vi "Stop Dependency.vi"(4 "timeout in ms (-1)":i32=-1, 6 "Destroy ref? (T)":bool=TRUE, 8 "error in (no error)":errorcluster, 9 "Name (ignored if reference valid)":string, 10 "Dependency Reference":refnum<class "SMO.lvclass">, 11 "SMO in":refnum<class "SMO.lvclass">) -> (0 "error out":errorcluster, 2 "Dependency Reference out":refnum<class "SMO.lvclass">, 3 "SMO out":refnum<class "SMO.lvclass">)   [LabVIEW 2021, in "smo.lvlib" / "SMO.lvclass"]
uses:
  SMO.lvclass
  SMO.lvclass/SMO.ctl
  Support/Attribute.Owner/Attribute.Owner.lvclass
  Typedefs/SMO Dependency Event--Enum.ctl
  Typedefs/SMO Dependency Event--Cluster.ctl
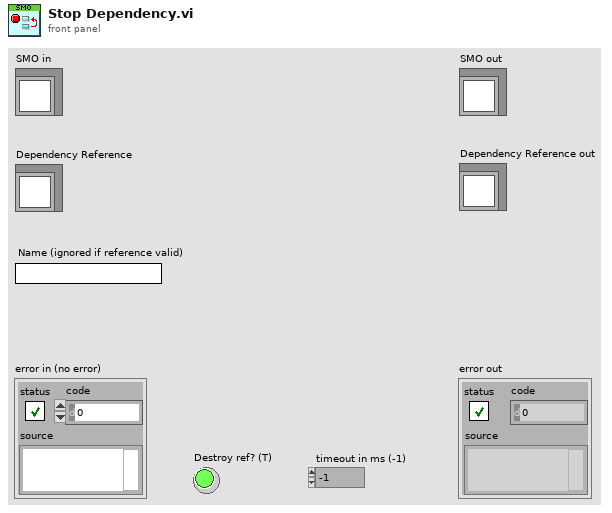
[diagram p1: front panel]
types:
  T1 = typedef "smo.lvlib/SMO.lvclass/SMO Dependency Event--Cluster.ctl" = cluster{"Name":string, "GUID":string, "Event":T2}
  T2 = typedef "smo.lvlib/SMO.lvclass/SMO Dependency Event--Enum.ctl" = enum16{"Added", "Removed", "Started", "Stopped"}
  T3 = typedef "smo.lvlib/SMO.lvclass/Protected Events.ctl" = cluster{"StopProcesses":refnum<user-event>, "AbortProcesses":refnum<user-event>, "Config Changed":refnum<user-event>, "Dependency":refnum<user-event>}
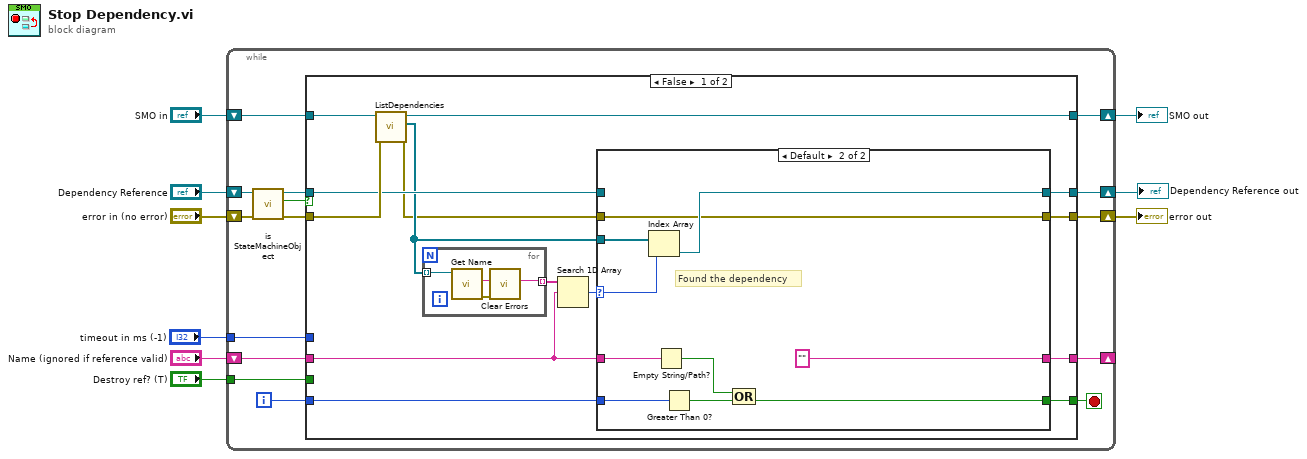
[diagram p0: block diagram]
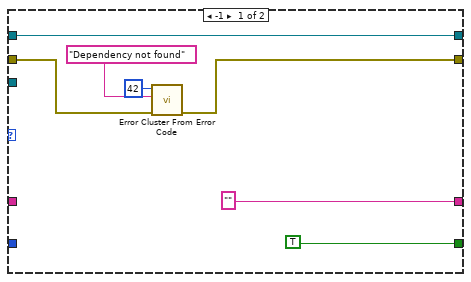
[diagram p2: hidden frame]
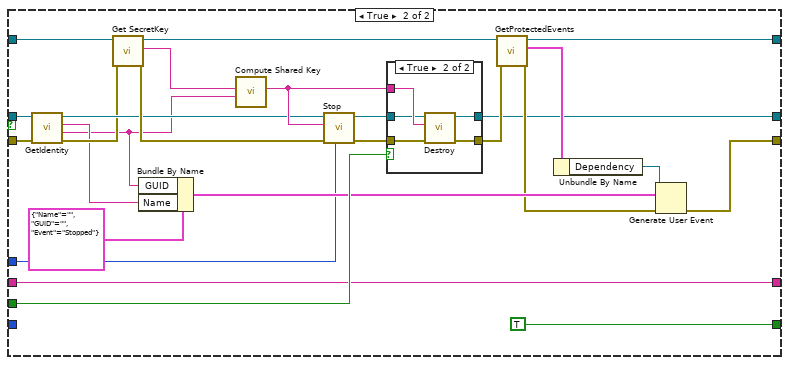
[diagram p3: hidden frame]
diagram:
  n1 = while {
    tunnel: "Destroy ref? (T)" -> [w15]
    shift-right: [w14] -> w2
    shift-left: "Dependency Reference" -> [w21]
    shift-right: [w24] -> w9
    shift-left: "error in (no error)" -> [w20]
    shift-right: [w22] -> w7
    shift-left: "SMO in" -> [w23]
    shift-right: [w11] -> _
    shift-left: "Name (ignored if reference valid)" -> [w16]
    tunnel: "timeout in ms (-1)" -> [w10]
    i -> [w12]
    stop <- w13 stop-if-true
    n2 = call "is StateMachineObject.vi"("error in (no error)"=w20, "SMO"=w21) -> ("error out"=w19:errorcluster, "is SMO?"=w18:bool, "SMO out"=w17:refnum<class "SMO.lvclass">)  [unwired: 7 in]
    n3 = case shown="False" w18 {
      tunnel: [w34 w69] -> w24
      tunnel: w23 -> [w38 w84]
      tunnel: [w26 w67] -> w22
      tunnel: w19 -> [w37 w61]
      tunnel: w17 -> [w32 w64]
      tunnel: w16 -> [w27 w76]
      tunnel: w15 -> [_ w78]
      tunnel: [w33 w66] -> w14
      tunnel: [w31 TRUE] -> w13
      tunnel: w12 -> [w29 _]
      tunnel: [w28 w76] -> w11
      tunnel: w10 -> [_ w65]
      frame False {
        n4 = call "ListDependencies.vi"("error in (no error)"=w37, "SMO in"=w38) -> ("error out"=w25:errorcluster, "[Dependencies]"=w30:refnum<class "SMO.lvclass">[], "SMO out"=w26:refnum<class "SMO.lvclass">)  [unwired: 6 in, 1 out]
        n5 = for {
          tunnel: w30 -> [w58] mode=indexing
          tunnel: [w57] -> w36 mode=indexing
          n6 = call "Get Name.vi"("SMO"=w58) -> ("error out"=w56:errorcluster, "Name"=w57:string)  [unwired: 6 in, 3 out]
          n7 = call <vilib>:"Clear Errors.vi"("error in (no error)"=w56) -> ()  [unwired: 5 in, 2 out]
        }
        n8 = Search 1D Array(1D array=w36, element=w27) -> (index of element=w35:i32)  [unwired: 1 in]
        n9 = case shown="Default" w35 {
          selector: w35 -> [_ w52]
          tunnel: [w42 w53] -> w34
          tunnel: w25 -> [w43 w53]
          tunnel: [w45 w54] -> w33
          tunnel: w32 -> [w45 _]
          tunnel: [TRUE w46] -> w31
          tunnel: w30 -> [_ w55]
          tunnel: w29 -> [_ w51]
          tunnel: ["" ("error message (\"\")") "" ("error message (\"\")")] -> w28
          tunnel: w27 -> [_ w49]
          frame -1 {
            n10 = call <vilib>:"Error Cluster From Error Code.vi"("error in (no error)"=w43, "error message (\"\")"="Dependency not found" ("error message (\"\")"), "error code (0)"=42) -> ("error out"=w42:errorcluster)  [unwired: 6 in]
          }
          frame Default {
            # "Found the dependency"
            n11 = Index Array(array=w55, index=w52) -> (element=w54:refnum<class "SMO.lvclass">)
            n12 = Empty String/Path?(string/path=w49) -> (empty?=w48:bool)
            n13 = Greater Than 0?(x=w51) -> (x > 0?=w47:bool)
            n14 = Compound Arithmetic op=OR(w48, w47) -> (w46:bool)
          }
        }
      }
      frame True {
        n15 = call "GetIdentity.vi"("error in (no error)"=w61, "SMO in"=w64) -> ("error out"=w62:errorcluster, "GUID"=w59:string, "Name"=w60:string, "SMO out"=w63:refnum<class "SMO.lvclass">)  [unwired: 6 in]
        n16 = call "Get SecretKey.vi"("error in (no error)"=w62, "SMO"=w84) -> ("error out"=w82:errorcluster, "SecretKey"=w83:string, "SMO out"=w68:refnum<class "SMO.lvclass">)  [unwired: 7 in]
        n17 = Bundle By Name(cluster=T1 {"Name"="", "GUID"="", "Event"=enum."Stopped"} ("Dependency Event"), "GUID"=w59, "Name"=w60) -> (w73:T1)
        n18 = call "Compute Shared Key.vi"("GUID"=w59, "SecretKey"=w83) -> ("Shared Key"=w79:string)  [unwired: 9 in]
        n19 = call "Stop.vi"("timeout in ms (-1)"=w65, "error in (no error)"=w82, "Shared Key"=w79, "SMO"=w63) -> ("error out"=w80:errorcluster, "SMO out"=w81:refnum<class "SMO.lvclass">)  [unwired: 6 in]
        n20 = case shown="True" w78 {
          tunnel: w81 -> [w86 w87]
          tunnel: w80 -> [w85 w90]
          tunnel: w79 -> [_ w89]
          tunnel: [w85 w88] -> w74
          tunnel: [w86 w87] -> w66
          frame False {
          }
          frame True {
            n21 = call "Destroy.vi"("error in (no error)"=w90, "Shared Key"=w89, "SMO"=w87) -> ("error out"=w88:errorcluster)  [unwired: 8 in]
          }
        }
        n22 = call "GetProtectedEvents.vi"("error in (no error)"=w74, "SMO"=w68) -> ("error out"=w70:errorcluster, "SMO Protected Events"=w72:T3, "SMO out"=w67:refnum<class "SMO.lvclass">)  [unwired: 7 in]
        n23 = Unbundle By Name(w72) -> ("Dependency"=w71:refnum<user-event>)
        n24 = Generate User Event(user event=w71, event data cluster=w73, error in=w70) -> (error out=w69:errorcluster)  [unwired: 1 in, 1 out]
      }
    }
  }
  "error out" <- w9
  "SMO out" <- w7
  "Dependency Reference out" <- w2
